vi "Do_ADAM_channel.vi"(4 "Scan Period":dbl format="%.2f", 5 "Previous Scan Value":dbl format="%.2f", 6 "Present scan array":dbl[](array[numeric]) format="%.2f", 7 "Value to Output":dbl format="%.2f", 8 "Ch Description":T1 {"Duty" format="%.0b"; "D" format="%#_5g"; "C" format="%#_5g"; "B" format="%#_5g"; "A" format="%#_5g"}, 9 "Ch names":string[](array[string])) -> (0 "Scan comment":string, 1 "Output":dbl format="%.3f")   [LabVIEW 2013]
uses:
  ADAM Client/Sub VIs/ADAM Controls/Ch_description_ADAM.ctl
  ADAM Client/Sub VIs/ADAM Controls/Module_type_ADAM.ctl
  ADAM Client/Sub VIs/ADAM Controls/Function_ADAM.ctl
  ADAM Client/Sub VIs/ADAM Controls/Channel_State.ctl
  ADAM Client/Sub VIs/ADAM Controls/Calib_type_ADAM.ctl
  ADAM Client/Sub VIs/ADAM Controls/Address.ctl
  ADAM Serial/Instrument drivers/Arduino/ctls_and_globals/Arduino tx msg cluster.ctl
  ADAM Client/Sub VIs/ADAM Controls/Remember_value_mode.ctl
  ADAM Client/Sub VIs/ADAM Controls/Search_mode.ctl
  Anemometry/Anemometry Sub Vis/Controls/In_Range.ctl
  Anemometry/Anemometry Sub Vis/Globals/Gas_management_global.vi
  ADAM_Global.vi
  Anemometry/Anemometry Sub Vis/Globals/Constants_global.vi
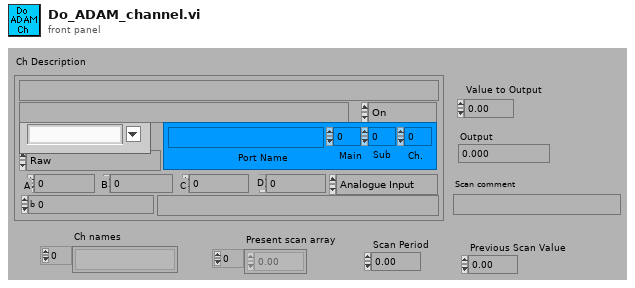
[diagram p1: front panel]
types:
  T1 = typedef "Ch_description_ADAM.ctl" = cluster{"Ch Name":string, "Type":T2, "Function":T3, "Ch State":T4, "Calibration type":T5, "A":dbl, "B":dbl, "C":dbl, "D":dbl, "Comments":string, "Address":T6, "String":string, "Duty":u16}
  T2 = typedef "Module_type_ADAM.ctl" = string
  T3 = typedef "Function_ADAM.ctl" = enum16{"Analogue Input", "Digital Input", "Event counter", "Event rate", "Analogue Output", "Digital Output", "Relay Output"}
  T4 = typedef "Channel_State.ctl" = enum16{"On", "Off", "Always On", "Always Off"}
  T5 = typedef "Calib_type_ADAM.ctl" = enum16{"Raw", "Bx + A", "Cx^2 + Bx + A", "Dx^3 + Cx^2 + Bx + A", "In Band", "Hi-Tec Q", "Hi-Tec M_dot", "Text"}
  T6 = typedef "Address.ctl" = cluster{"Main":i32, "Ch.":i32, "Sub":i32, "Port Name":string}
  T7 = typedef "Remember_value_mode.ctl" = enum16{"Read only", "Read and Write"}
  T8 = typedef "Search_mode.ctl" = enum16{"Between times", "All Times"}
  T9 = typedef "In_Range.ctl" = enum16{"%", "±", "% & ±"}
  T10 = typedef "Arduino tx msg cluster.ctl" = cluster{"dest":u8, "A/D":string, "R/W":string, "chan":u8, "val (float)":sgl}
  T11 = typedef "Valco_valve_ph.ctl" = u16
  T12 = cluster{"Centre Times":dbl[], "Output array":dbl[]}
  T13 = cluster{"Centre Times":dbl[], "Output array":dbl[]}[]
  T14 = typedef "LVDateTimeRec.ctl" = cluster{"fractional second":dbl, "second":i32, "minute":i32, "hour":i32, "day of month":i32, "month":i32, "year":i32, "day of week":i32, "day of year":i32, "DST":i32}
  T15 = typedef "Client_State_Cluster.ctl" = cluster{"Client Name":string, "Traverse level State":T16, "People to Email":string[], "Next Contact Time":dbl}
  T16 = typedef "Traverse_Level_State.ctl" = enum16{"Running", "Complete"}
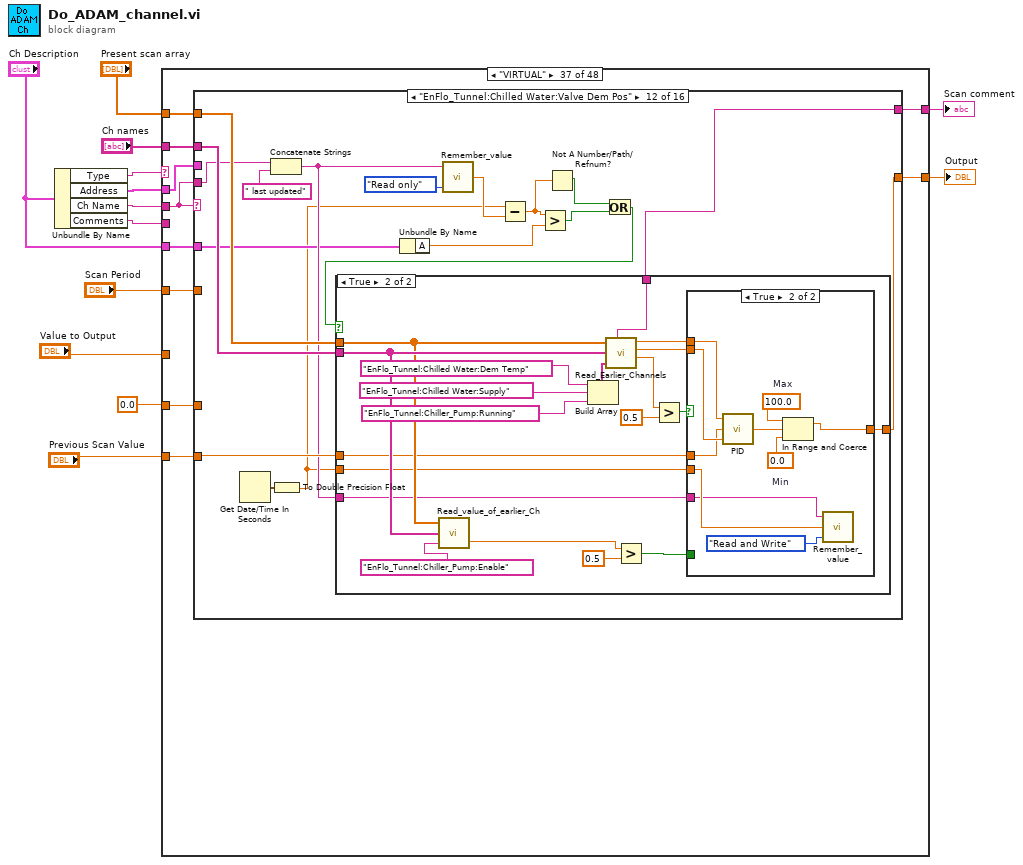
[diagram p0: block diagram]
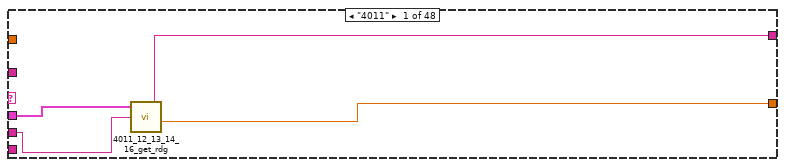
[diagram p2: hidden frame]
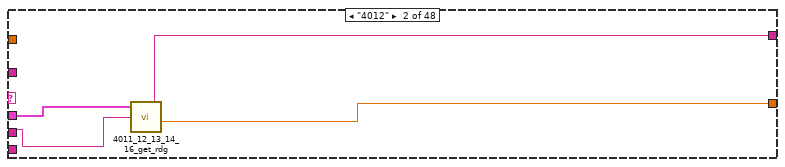
[diagram p3: hidden frame]
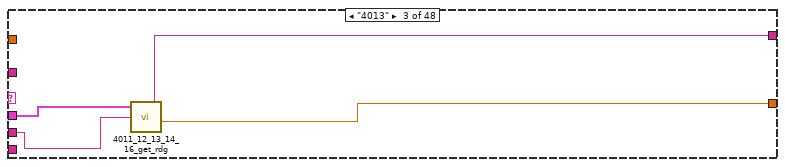
[diagram p4: hidden frame]
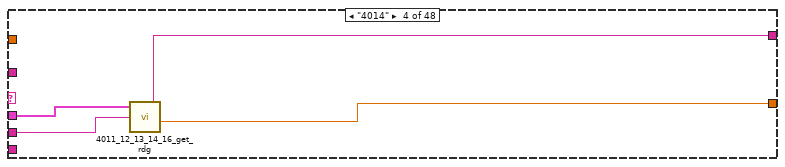
[diagram p5: hidden frame]
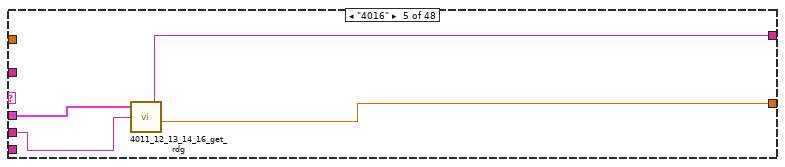
[diagram p6: hidden frame]
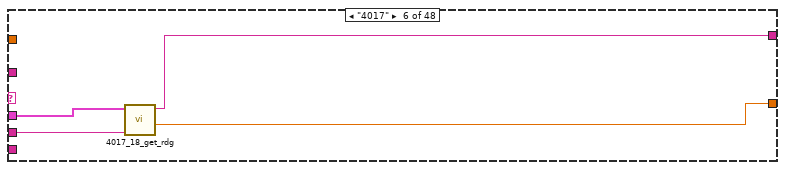
[diagram p7: hidden frame]
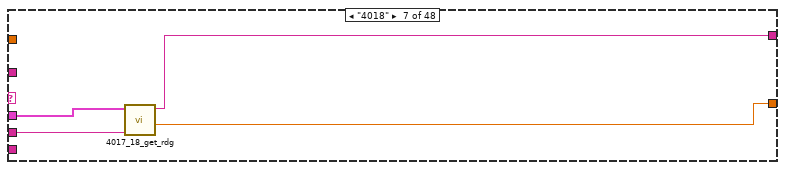
[diagram p8: hidden frame]
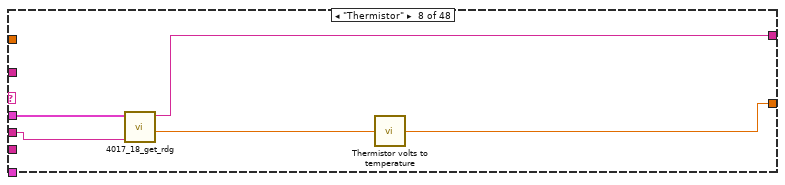
[diagram p9: hidden frame]
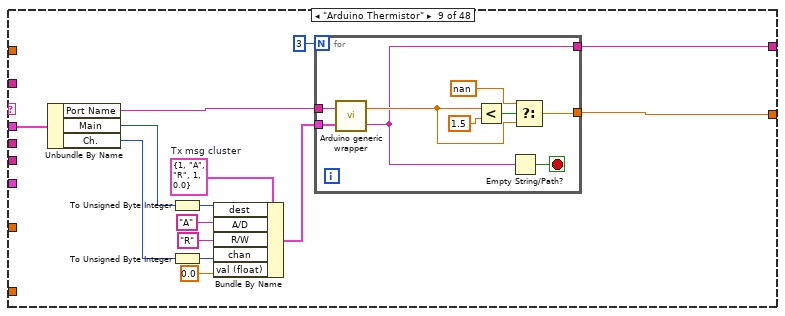
[diagram p10: hidden frame]
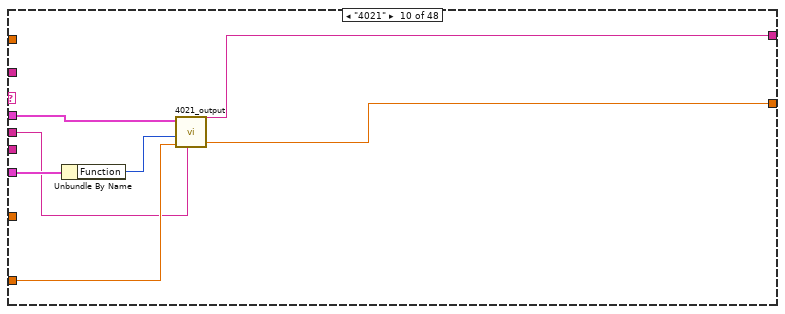
[diagram p11: hidden frame]
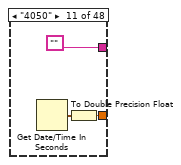
[diagram p12: hidden frame]
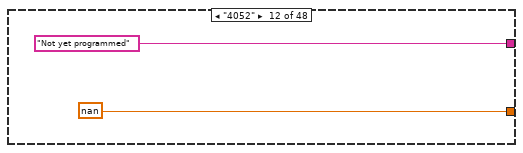
[diagram p13: hidden frame]
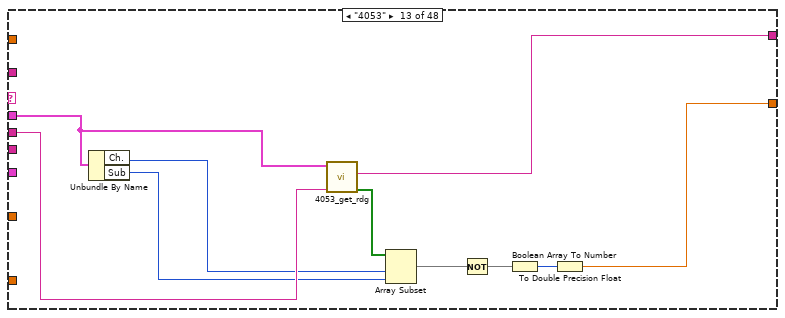
[diagram p14: hidden frame]
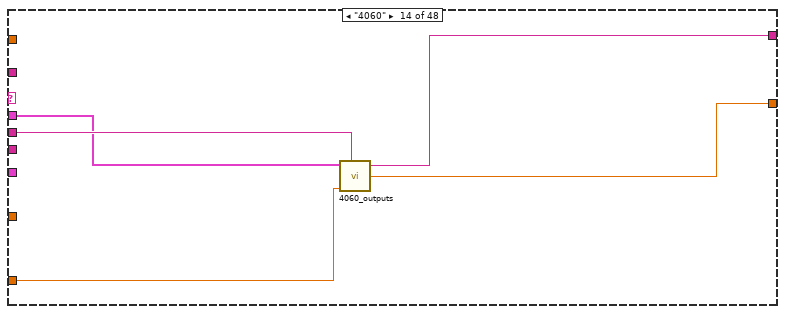
[diagram p15: hidden frame]
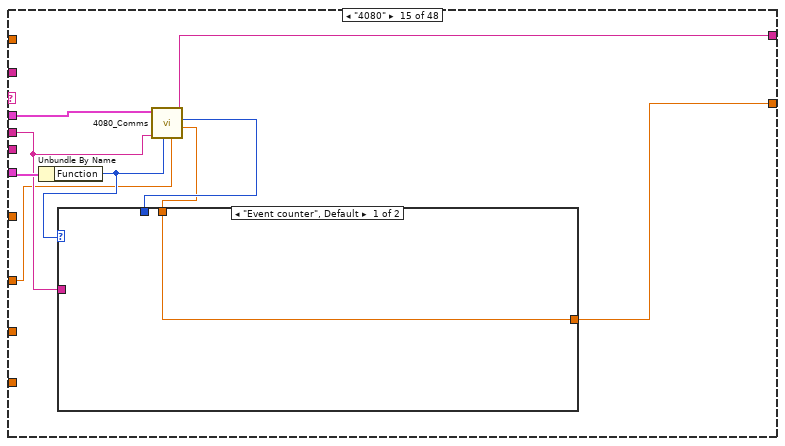
[diagram p16: hidden frame]
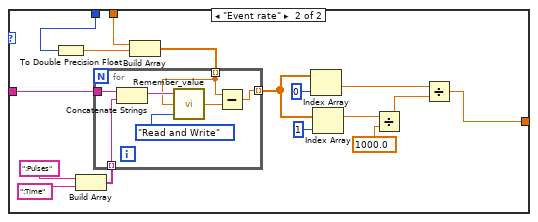
[diagram p17: hidden frame]
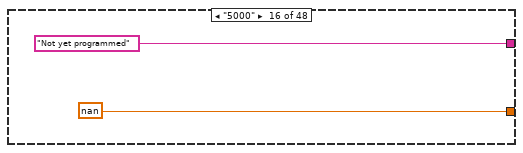
[diagram p18: hidden frame]
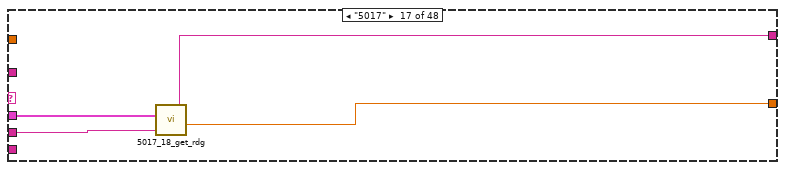
[diagram p19: hidden frame]
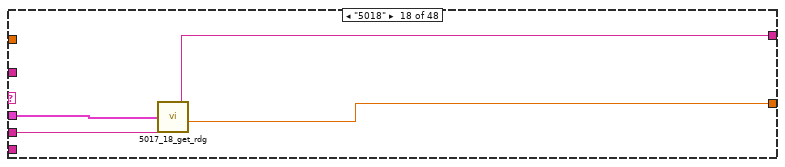
[diagram p20: hidden frame]
diagram:
  n1 = Unbundle By Name("Ch Description") -> ("Type"=w11:T2, "Address"=w10:T6, "Ch Name"=w2:string, "Comments"=w7:string)
  n2 = case shown="\"VIRTUAL\"" w11 {
    tunnel: [w16 w20 w24 w28 w32 w36 w40 w42 w48 w75 w78 nan w85 w94 w103 nan w133 w137 w142 w148 w156 w177 w199 w218 nan w286 w288 w304 w327 w366 nan w378 w409 w414 w415 w518 w542 w978 w980 w984 w989 w1001 w1035 w1061 w1071 w1076 w1086 0.0 ("Output")] -> w8
    tunnel: [w17 w21 w25 w29 w33 w37 w41 w46 w49 w76 "" "Not yet programmed" w90 w95 w105 "Not yet programmed" w134 w138 w145 w149 w155 w178 w200 w220 "Not yet programmed" w285 w289 w303 w319 w367 "Not yet programmed" w377 w410 w413 w436 w520 w541 "" "" w985 "" "" w1024 "" w1072 w1075 "Crazy time based random number!" "Warning; unmatched case in Do_ADAM_channel" ("Status note")] -> w5
    tunnel: w10 -> [w14 w18 w22 w26 w30 w34 w38 w44 w60 w70 _ _ w82 w93 w97 _ w135 w139 w146 w150 w154 w179 w201 w222 _ w283 w287 w306 w324 w372 _ _ w408 w411 _ _ w533 _ _ _ _ _ _ w1070 w1074 _ _ _]
    tunnel: "Ch Description" -> [_ _ _ _ _ _ _ _ _ w74 _ _ _ _ w104 _ _ _ _ _ w153 w176 w198 w221 _ _ _ _ _ _ _ w383 _ _ w441 _ w535 _ w981 w986 _ _ _ _ _ w1077 _ _]
    tunnel: w2 -> [w15 w19 w23 w27 w31 w35 w39 w45 _ w71 _ _ w91 w96 w100 _ w132 w136 w140 w147 w151 w173 w195 w219 _ w284 _ w305 w320 w371 _ _ _ w412 _ _ w538 _ _ _ _ w997 w1031 _ w1073 _ _ _]
    tunnel: "Ch names" -> [_ _ _ _ _ _ _ _ _ _ _ _ _ _ _ _ _ _ _ _ _ _ _ _ _ _ _ _ _ _ _ w384 _ _ w440 w525 w540 _ _ w987 _ _ _ _ _ _ _ _]
    tunnel: "Present scan array" -> [_ _ _ _ _ _ _ _ _ _ _ _ _ _ _ _ _ _ _ _ _ _ _ _ _ _ _ _ _ _ _ w381 _ _ w438 w524 w539 _ _ w988 _ _ _ _ _ _ _ _]
    tunnel: w7 -> [_ _ _ _ _ _ _ _ _ _ _ _ _ _ _ _ _ _ _ _ _ _ _ _ _ _ _ _ _ _ _ w376 _ _ w442 w523 _ _ _ _ _ _ _ _ _ _ _ _]
    tunnel: "Value to Output" -> [_ _ _ _ _ _ _ _ _ w72 _ _ _ w92 w98 _ _ _ w141 _ w152 w174 w196 w217 _ _ _ w302 w328 _ _ w382 _ _ _ _ _ _ _ _ _ _ _ w1065 _ _ _ _]
    tunnel: "Scan Period" -> [_ _ _ _ _ _ _ _ _ _ _ _ _ _ _ _ _ _ _ _ _ _ _ _ _ _ _ _ _ _ _ w379 _ _ _ _ w537 _ _ _ _ _ _ _ _ _ _ _]
    tunnel: "Previous Scan Value" -> [_ _ _ _ _ _ _ _ _ _ _ _ _ _ _ _ _ _ _ _ _ _ _ _ _ _ _ _ _ _ _ w380 _ _ w416 _ w536 w978 _ _ w989 _ _ _ _ _ _ _]
    tunnel: 0.0 -> [_ _ _ _ _ _ _ _ _ _ _ _ _ _ _ _ _ _ _ _ _ _ _ _ _ _ _ _ _ _ _ _ _ _ _ _ w534 _ _ _ _ _ _ _ _ _ _ _]
    frame "4011" {
      n3 = call "4011_12_13_14_16_get_rdg.vi"("Address"=w14, "Channel Name"=w15) -> ("Comment"=w17:string, "Reading"=w16:dbl)  [unwired: 1 in, 2 out]
    }
    frame "4012" {
      n4 = call "4011_12_13_14_16_get_rdg.vi"("Address"=w18, "Channel Name"=w19) -> ("Comment"=w21:string, "Reading"=w20:dbl)  [unwired: 1 in, 2 out]
    }
    frame "4013" {
      n5 = call "4011_12_13_14_16_get_rdg.vi"("Address"=w22, "Channel Name"=w23) -> ("Comment"=w25:string, "Reading"=w24:dbl)  [unwired: 1 in, 2 out]
    }
    frame "4014" {
      n6 = call "4011_12_13_14_16_get_rdg.vi"("Address"=w26, "Channel Name"=w27) -> ("Comment"=w29:string, "Reading"=w28:dbl)  [unwired: 1 in, 2 out]
    }
    frame "4016" {
      n7 = call "4011_12_13_14_16_get_rdg.vi"("Address"=w30, "Channel Name"=w31) -> ("Comment"=w33:string, "Reading"=w32:dbl)  [unwired: 1 in, 2 out]
    }
    frame "4017" {
      n8 = call "4017_18_get_rdg.vi"("Channel Name"=w35, "Address"=w34) -> ("Reading"=w36:dbl, "Comment"=w37:string)  [unwired: 2 in, 2 out]
    }
    frame "4018" {
      n9 = call "4017_18_get_rdg.vi"("Channel Name"=w39, "Address"=w38) -> ("Reading"=w40:dbl, "Comment"=w41:string)  [unwired: 2 in, 2 out]
    }
    frame "Thermistor" {
      n10 = call "4017_18_get_rdg.vi"("Channel Name"=w45, "Address"=w44) -> ("Reading"=w43:dbl, "Comment"=w46:string)  [unwired: 2 in, 2 out]
      n11 = call "Thermistor volts to temperature.vi"("V2 (V)"=w43) -> ("Temperature (degC)"=w42:dbl)
    }
    frame "Arduino Thermistor" {
      w54 = T10 {"dest"=1, "A/D"="A", "R/W"="R", "chan"=1, "val (float)"=0.0}  # Tx msg cluster
      n12 = Unbundle By Name(w60) -> ("Port Name"=w51:string, "Main"=w52:i32, "Ch."=w53:i32)
      n13 = To Unsigned Byte Integer(number=w52) -> (unsigned 8bit integer=w59:u8)
      n14 = To Unsigned Byte Integer(number=w53) -> (unsigned 8bit integer=w57:u8)
      n15 = Bundle By Name(cluster=w54, "dest"=w59, "A/D"="A", "R/W"="R", "chan"=w57, "val (float)"=sgl 0.0) -> (w50:T10)
      n16 = for {
        N: 3 -> [_]
        tunnel: w51 -> [w69]
        tunnel: w50 -> [w68]
        tunnel: [w61] -> w49
        tunnel: [w67] -> w48
        stop <- w62 stop-if-true
        n17 = call "Arduino generic wrapper.vi"("Tx msg cluster"=w68, "Port name"=w69) -> ("Scan comment"=w61:string, "Output"=w66:dbl)
        n18 = Less?(x=w66, y=1.5) -> (x < y?=w64:bool)
        n19 = Empty String/Path?(string/path=w61) -> (empty?=w62:bool)
        n20 = Select(t=nan ("f"), s=w64, f=w66) -> (s? t:f=w67:dbl)
      }
    }
    frame "4021" {
      n21 = Unbundle By Name(w74) -> ("Function"=w73:T3)
      n22 = call "4021_output.vi"("Address"=w70, "Function"=w73, "Set to:"=w72, "Channel Name"=w71) -> ("Comment"=w76:string, "Reading"=w75:dbl)  [unwired: 1 in, 1 out]
    }
    frame "4050" {
      n23 = Get Date/Time In Seconds() -> (seconds since 1Jan1904=w77:timestamp)
      n24 = To Double Precision Float(number=w77) -> (double precision float=w78:dbl)
    }
    frame "4052" {
    }
    frame "4053" {
      n25 = Unbundle By Name(w82) -> ("Ch."=w83:i32, "Sub"=w89:i32)
      n26 = call "4053_get_rdg.vi"("Channel Name"=w91, "Address"=w82) -> ("Boolean array"=w88:bool[], "Comment"=w90:string)  [unwired: 2 in, 2 out]
      n27 = Array Subset(array=w88, index=w83, length=w89) -> (w87:bool[])
      n28 = Not(x=w87) -> (.not. x?=w84:bool[])
      n29 = Boolean Array To Number(Boolean array=w84) -> (number=w86:u32)
      n30 = To Double Precision Float(number=w86) -> (double precision float=w85:dbl)
    }
    frame "4060" {
      n31 = call "4060_outputs.vi"("Address"=w93, "Value to Output"=w92, "Channel Name"=w96) -> ("Comment"=w95:string, "Reading"=w94:dbl)  [unwired: 2 in, 1 out]
    }
    frame "4080" {
      n32 = Unbundle By Name(w104) -> ("Function"=w99:T3)
      n33 = call "4080_Comms.vi"("Value to display"=w98, "Function"=w99, "Channel Name"=w100, "Address"=w97) -> ("Reading"=w101:dbl, "millisecond timer value"=w102:u32, "Comment"=w105:string)  [unwired: 2 in, 1 out]
      n34 = case shown="\"Event counter\", Default" w99 {
        tunnel: w100 -> [_ w122]
        tunnel: w102 -> [_ w115]
        tunnel: [w106 w107] -> w103
        tunnel: w101 -> [w106 w116]
        frame "Event counter", Default {
        }
        frame "Event rate" {
          n35 = To Double Precision Float(number=w115) -> (double precision float=w114:dbl)
          n36 = Build Array(":Pulses", ":Time") -> (w117:string[])
          n37 = Build Array(w116, w114) -> (w113:dbl[])
          n38 = for {
            tunnel: w122 -> [w126]
            tunnel: [w127] -> w110 mode=indexing
            tunnel: w117 -> [w124] mode=indexing
            tunnel: w113 -> [w123] mode=indexing
            n39 = Concatenate Strings(w126, w124) -> (w125:string)
            n40 = call "Remember_value.vi"("Mode"=Remember_value_mode."Read and Write", "Input Value"=w123, "Ch name"=w125) -> ("Output Value"=w128:dbl)
            n41 = Subtract(x=w123, y=w128) -> (x-y=w127:dbl)
          }
          n42 = Index Array(array=w110, index=0) -> (element=w108:dbl)
          n43 = Index Array(array=w110, index=1) -> (element=w109:dbl)
          n44 = Divide(x=w109, y=1000.0) -> (x/y=w120:dbl)
          n45 = Divide(x=w108, y=w120) -> (x/y=w107:dbl)
        }
      }
    }
    frame "5000" {
    }
    frame "5017" {
      n46 = call "5017_18_get_rdg.vi"("Address (all reqd.)"=w135, "Channel Name"=w132) -> ("Comment"=w134:string, "Reading"=w133:dbl)  [unwired: 3 out]
    }
    frame "5018" {
      n47 = call "5017_18_get_rdg.vi"("Address (all reqd.)"=w139, "Channel Name"=w136) -> ("Comment"=w138:string, "Reading"=w137:dbl)  [unwired: 3 out]
    }
    frame "5024" {
      n48 = call "5024_set_output.vi"("Set to:"=w141, "Address (all reqd.)"=w146, "Channel Name"=w140) -> ("Comment"=w145:string, "Good Reply"=w143:bool)  [unwired: 2 out]
      n49 = Select(t=w141, s=w143, f=nan) -> (s? t:f=w142:dbl)
    }
    frame "5051" {
      n50 = call "5051_56_get_inputs.vi"("Address (Main, Sub reqd.)"=w150, "Channel Name"=w147) -> ("Comment"=w149:string, "Single output"=w148:dbl)  [unwired: 3 out]
    }
    frame "5056" {
      n51 = Unbundle By Name(w153) -> ("Function"=w157:T3)
      n52 = case shown="\"Digital Input\"" w157 {
        tunnel: w154 -> [_ w163 w172]
        tunnel: ["This function is not available" w164 w170] -> w155
        tunnel: [nan ("A") w161 w167] -> w156
        tunnel: w152 -> [_ _ w166]
        tunnel: w151 -> [_ w160 w165]
        frame "Analogue Input", Default {
        }
        frame "Digital Input" {
          # "Readback value"
          n53 = call "5060_check_outputs.vi"("Address (Main, Sub reqd.)"=w163, "Channel Name"=w160) -> ("Comment"=w164:string, "Single Channel"=w162:i16)  [unwired: 3 out]
          n54 = To Double Precision Float(number=w162) -> (double precision float=w161:dbl)
        }
        frame "Relay Output" {
          # "Sets single o/p channel"
          n55 = Greater Than 0?(x=w166) -> (x > 0?=w171:bool)
          n56 = call "5056_60_set_single_output.vi"("Channel Name"=w165, "Address (all reqd.)"=w172, "Set state:"=w171) -> ("Comment"=w170:string, "Good Reply"=w169:bool)  [unwired: 2 out]
          n57 = Select(t=w166, s=w169, f=nan) -> (s? t:f=w167:dbl)
        }
      }
    }
    frame "5060" {
      n58 = Unbundle By Name(w176) -> ("Function"=w175:T3)
      n59 = case shown="\"Relay Output\"" w175 {
        tunnel: w179 -> [_ w185 w194]
        tunnel: ["This function is not available" w186 w192] -> w178
        tunnel: [nan ("A") w183 w189] -> w177
        tunnel: w174 -> [_ _ w188]
        tunnel: w173 -> [_ w182 w187]
        frame "Analogue Input", Default {
        }
        frame "Digital Input" {
          # "Readback value"
          n60 = call "5060_check_outputs.vi"("Address (Main, Sub reqd.)"=w185, "Channel Name"=w182) -> ("Comment"=w186:string, "Single Channel"=w184:i16)  [unwired: 3 out]
          n61 = To Double Precision Float(number=w184) -> (double precision float=w183:dbl)
        }
        frame "Relay Output" {
          # "Sets single o/p channel"
          n62 = Greater Than 0?(x=w188) -> (x > 0?=w193:bool)
          n63 = call "5056_60_set_single_output.vi"("Channel Name"=w187, "Address (all reqd.)"=w194, "Set state:"=w193) -> ("Comment"=w192:string, "Good Reply"=w191:bool)  [unwired: 2 out]
          n64 = Select(t=w188, s=w191, f=nan) -> (s? t:f=w189:dbl)
        }
      }
    }
    frame "6060" {
      n65 = Unbundle By Name(w198) -> ("Function"=w197:T3)
      n66 = case shown="\"Digital Input\"" w197 {
        tunnel: w201 -> [_ w207 w216]
        tunnel: ["This function is not available" w208 w214] -> w200
        tunnel: [nan ("A") w205 w211] -> w199
        tunnel: w196 -> [_ _ w210]
        tunnel: w195 -> [_ w204 w209]
        frame "Analogue Input", Default {
        }
        frame "Digital Input" {
          n67 = call "6060_read_all_I-O.vi"("Address (Main, Sub reqd.)"=w207, "Channel Name"=w204) -> ("Comment"=w208:string, "Single Input Channel"=w206:i16)  [unwired: 3 out]
          n68 = To Double Precision Float(number=w206) -> (double precision float=w205:dbl)
        }
        frame "Relay Output" {
          # "Sets single o/p channel"
          n69 = Greater Than 0?(x=w210) -> (x > 0?=w215:bool)
          n70 = call "6060_set_single_output.vi"("Channel Name"=w209, "Address (Main, Ch requd.)"=w216, "Set state:"=w215) -> ("Comment"=w214:string, "Good Reply"=w213:bool)  [unwired: 2 out]
          n71 = Select(t=w210, s=w213, f=nan) -> (s? t:f=w211:dbl)
        }
      }
    }
    frame "Tracker" {
      n72 = while {
        tunnel: w222 -> [w246]
        tunnel: w221 -> [w245]
        tunnel: [w239] -> w220
        tunnel: w219 -> [w238]
        tunnel: [w232] -> w218
        tunnel: w217 -> [w231]
        i -> [w228]
        stop <- w225 continue-if-true
        n73 = Unbundle By Name(w245) -> ("Function"=w244:T3)
        n74 = Unbundle By Name(w246) -> ("Port Name"=w243:string, "Ch."=w234:i32, "Main"=w242:i32, "Sub"=w241:i32)
        n75 = case shown="\"Analogue Output\"" w244 {
          tunnel: [enum16{"Set", "Read"}."Set" ("Set") enum16{"Set", "Read"}."Set" ("Set") enum16{"Set", "Read"}."Set" ("Set") enum16{"Set", "Read"}."Set" ("Set") enum16{"Set", "Read"}."Set" ("Set") enum16{"Set", "Read"}."Read" ("Set") enum16{"Set", "Read"}."Read" ("Set")] -> w229
          tunnel: [enum16{"Logic", "Analogue"}."Analogue" ("Analogue") enum16{"Logic", "Analogue"}."Logic" ("Analogue") enum16{"Logic", "Analogue"}."Logic" ("Analogue") enum16{"Logic", "Analogue"}."Logic" ("Analogue") enum16{"Logic", "Analogue"}."Logic" ("Analogue") enum16{"Logic", "Analogue"}."Logic" ("Analogue") enum16{"Logic", "Analogue"}."Analogue" ("Analogue")] -> w240
          frame "Analogue Output" {
          }
          frame "Digital Output" {
          }
          frame "Relay Output" {
          }
          frame "Event rate" {
          }
          frame "Event counter" {
          }
          frame "Digital Input" {
          }
          frame "Analogue Input" {
          }
        }
        n76 = call "TalkTracker.vi"("PORT NAME"=w243, "Set"=w229, "Channel Name"=w238, "Value to set"=w231, "MODULE ADDRESS"=w242, "LOCATION"=w234, "NO. LOCATIONS"=w241, "Analogue"=w240) -> ("Response"=w236:string, "Good Set?"=w223:bool, "Comment out"=w239:string)  [unwired: 1 in, 4 out]
        n77 = Match Pattern(string=w236, regular expression="\r\n") -> (before substring=w235:string)  [unwired: 4 out]
        n78 = case shown="\"Set\"" w229 {
          tunnel: w235 -> [_ w258]
          tunnel: [w250 w257] -> w233
          tunnel: w231 -> [w252 _]
          tunnel: nan ("Reading") -> [w251 w256]
          tunnel: [w249 w254] -> w226
          tunnel: [0 ("y") 1 ("y")] -> w224
          tunnel: w223 -> [w247 _]
          frame "Set" {
            n79 = Not(x=w247) -> (.not. x?=w249:bool)
            n80 = Select(t=w252, s=w247, f=w251) -> (s? t:f=w250:dbl)
          }
          frame "Read" {
            n81 = String Length(string=w258) -> (length=w260:i32)
            n82 = Fract/Exp String To Number(string=w258, default (0 dbl)=w256) -> (offset past number=w261:i32, number=w259:dbl)  [unwired: 2 out]
            n83 = Equal?(x=w260, y=w261) -> (x = y?=w255:bool)
            n84 = Not(x=w255) -> (.not. x?=w254:bool)
            n85 = Select(t=w259, s=w255, f=w256) -> (s? t:f=w257:dbl)
          }
        }
        n86 = case shown="0, Default" w234 {
          tunnel: w233 -> [w262 w265]
          tunnel: [w262 w263] -> w232
          frame 0, Default {
          }
          frame 283 {
            n87 = Equal To 0?(x=w265) -> (x = 0?=w266:bool)
            n88 = Select(t=nan ("Reading"), s=w266, f=w265) -> (s? t:f=w263:dbl)
          }
        }
        n89 = Less?(x=w228, y=w224) -> (x < y?=w227:bool)
        n90 = And(x=w226, y=w227) -> (x .and. y?=w225:bool)
      }
    }
    frame "WEST" {
    }
    frame "GILL" {
      n91 = call "Gill_get_rdg.vi"("Channel Name"=w284, "Address"=w283) -> ("Output"=w286:dbl, "Status note"=w285:string)  [unwired: 2 in, 2 out]
    }
    frame "ClimatronicsUDP" {
      n92 = call "ClimatronicsUDP_get_rdg.vi"("Address"=w287) -> ("Output"=w288:dbl, "Status note"=w289:string)  [unwired: 5 in]
    }
    frame "JEM" {
      n93 = Unbundle By Name(w306) -> ("Main"=w292:i32, "Ch."=w291:i32, "Port Name"=w301:string)
      n94 = case shown="0, Default" w291 {
        tunnel: [i16[] [-3, -2, -1, 0, 14, 29, 43, 57, 71, 86, 100] i16[] [0, 20, 40, 60, 80, 100, 120]] -> w295
        tunnel: [u8[] [10, 50, 80, 100, 120, 140, 160, 180, 200, 220, 240] u8[] [20, 50, 90, 130, 160, 200, 230]] -> w296
        frame 0, Default {
        }
        frame 1 {
        }
      }
      n95 = Add(x=w292, y=w291) -> (x+y=w290:i32)
      n96 = Threshold 1D Array(2:w302, 3:w295) -> (0:w298:dbl)  [unwired: 1 out]
      n97 = Round To Nearest(number=w298) -> (nearest integer value=w299:dbl)
      n98 = To Long Integer(number=w299) -> (32bit integer=w297:i32)
      n99 = Index Array(array=w296, index=w297) -> (element=w294:u8)
      n100 = call "DMX.vi"("Port Name"=w301, "DMX channel no."=w290, "Set value:"=w294, "Channel Name"=w305) -> ("error"=w300:bool)  [unwired: 2 out]
      n101 = Index Array(array=w295, index=w297) -> (element=w293:i16)
      n102 = case shown="False" w300 {
        tunnel: [w307 nan] -> w304
        tunnel: ["" "Comms Error"] -> w303
        tunnel: w293 -> [w309 _]
        frame False {
          n103 = To Double Precision Float(number=w309) -> (double precision float=w307:dbl)
        }
        frame True {
        }
      }
    }
    frame "VICI" {
      n104 = To Long Integer(number=w328) -> (32bit integer=w323:i32)
      n105 = Unbundle By Name(w324) -> ("Port Name"=w326:string, "Ch."=w325:i32)
      n106 = call "Valco_Valve_Position.vi"("Channel Name"=w320, "Valve Number"=w325, "Port Name"=w326, "Requested Posn."=w323) -> ("Error Message"=w318:string, "Achieved Posn."=w321:T11)  [unwired: 2 out]
      n107 = Empty String/Path?(string/path=w318) -> ()  [unwired: 1 out]
      n108 = case shown="True" TRUE {
        tunnel: w324 -> [w335 _]
        tunnel: w323 -> [w334 _]
        tunnel: [w333 w365] -> w322
        tunnel: w321 -> [_ w365]
        tunnel: w320 -> [w332 _]
        tunnel: [w331 w364] -> w319
        tunnel: w318 -> [_ w364]
        tunnel: w318 -> [w330 _]
        tunnel: "X10" ("Port Name") -> [w329 _]
        frame False {
          n109 = stacked-sequence {
            tunnel: w335 -> [_ _ _ _ _ w356]
            tunnel: w334 -> [_ _ _ _ _ w352]
            tunnel: [_ _ _ _ _ w355] -> w333
            tunnel: w332 -> [_ _ _ _ _ w354]
            tunnel: [_ _ _ _ _ w353] -> w331
            tunnel: w330 -> [_ w341 _ _ _ _]
            tunnel: w329 -> [w336 _ _ w344 _ _]
            frame #0 {
              w338 = 3 items=["-----", "A", "B", "C", "D", "E", "F", "G", "H", "I", "J", "K", "L", "M", "N", "O", "P"] ("House Code")
              n110 = call "X10control.vi"("Port Name"=w336, "Power Request (ON)"=FALSE, "House Code"=w338, "Unit No."=5) -> ()  [unwired: 6 out]
            }
            frame #1 {
              n111 = call "Server_Emails.vi"("Message"=w341, "Contact All clients?"=TRUE, "Subject"="Powering Down FID Valve" ("Error Type")) -> ()  [unwired: 2 in, 3 out]
            }
            frame #2 {
              n112 = Wait (ms)(milliseconds to wait=u32 20000) -> ()  [unwired: 1 out]
            }
            frame #3 {
              w346 = 3 items=["-----", "A", "B", "C", "D", "E", "F", "G", "H", "I", "J", "K", "L", "M", "N", "O", "P"] ("House Code")
              n113 = call "X10control.vi"("Port Name"=w344, "Power Request (ON)"=TRUE, "House Code"=w346, "Unit No."=5) -> ()  [unwired: 6 out]
            }
            frame #4 {
              n114 = Wait (ms)(milliseconds to wait=u32 5000) -> ()  [unwired: 1 out]
            }
            frame #5 {
              n115 = Build Array(1 ("element"), 2 ("element"), w352) -> (w349:i32[])
              n116 = for {
                tunnel: w356 -> [w361]
                tunnel: [w360] -> w355
                tunnel: w354 -> [w359]
                tunnel: [w358] -> w353
                tunnel: w349 -> [w357] mode=indexing
                n117 = Unbundle By Name(w361) -> ("Port Name"=w362:string, "Ch."=w363:i32)
                n118 = call "Valco_Valve_Position.vi"("Channel Name"=w359, "Valve Number"=w363, "Port Name"=w362, "Requested Posn."=w357) -> ("Error Message"=w358:string, "Achieved Posn."=w360:T11)  [unwired: 2 out]
              }
            }
          }
        }
        frame True {
        }
      }
      n119 = To Double Precision Float(number=w322) -> (double precision float=w327:dbl)
    }
    frame "Vaisala" {
      n120 = Unbundle By Name(w372) -> ("Main"=w368:i32, "Ch."=w369:i32, "Port Name"=w370:string)
      n121 = call "HMP231.vi"("Channel Name"=w371, "Port Name"=w370, "Channel"=w369, "Address"=w368) -> ("Output"=w366:dbl, "Status note"=w367:string)  [unwired: 2 out]
    }
    frame "DRUCK" {
    }
    frame "Run VI Named:" {
      n122 = Current VI's Path() -> (path=w393:path)
      n123 = Strip Path(path=w393) -> (stripped path=w394:path)  [unwired: 1 out]
      n124 = call <vilib>:"Trim Whitespace.vi"("string"=w376) -> ("trimmed string"=w375:string)  [unwired: 1 in]
      n125 = Strip Path(path=w394) -> (stripped path=w395:path)  [unwired: 1 out]
      n126 = Build Path(base path=w395, name or relative path="Run_vi_named") -> (appended path=w397:path)
      n127 = Build Path(base path=w397, name or relative path=w375) -> (appended path=w392:path)
      n128 = Open VI Reference(type specifier VI Refnum (for type only)=refnum<vi> refnum, vi path=w392) -> (vi reference=w388:refnum<vi>, error out=w387:errorcluster)  [unwired: 1 in, 3 out]
      n129 = property class="VI Interface Type 0"(reference=w388, error in=w387) -> (reference out=w390:refnum<vi>, error out=w389:errorcluster, "Front Panel Window:Open"=w391:bool)
      n130 = case shown="False" w391 {
        tunnel: w390 -> [w405 w407]
        tunnel: w389 -> [w404 w406]
        tunnel: [w403 w407] -> w386
        tunnel: [w401 w406] -> w385
        frame False {
          n131 = property class="VI Interface Type 0"(reference=w405, error in=w404, "Front Panel Window:Open"=TRUE) -> (reference out=w403:refnum<vi>, error out=w401:errorcluster)
        }
        frame True {
        }
      }
      n132 = call-by-ref "?"(reference=w386, error in=w385, "Scan Period"=w379, "Previous Scan Value"=w380, "Present scan array"=w381, "Value to Output"=w382, "Ch Description"=w383, "Ch names"=w384) -> (reference out=w399:refnum<vi>, error out=w400:errorcluster, "Scan comment"=w377:string, "Output"=w378:dbl)  [unwired: 2 in]
      n133 = Close Reference(reference=w399, error in (no error)=w400) -> ()  [unwired: 1 out]
    }
    frame "IR2100" {
      n134 = call "IR2100_get_rdg.vi"("Address"=w408) -> ("Comment"=w410:string, "Reading"=w409:dbl)  [unwired: 2 in, 2 out]
    }
    frame "PPT" {
      n135 = call "PPT_get_rdg.vi"("Channel Name"=w412, "Address"=w411) -> ("Reading"=w414:dbl, "Comment"=w413:string)  [unwired: 2 in, 2 out]
    }
    frame "Comparator" {
      # "A Warn if above this value\nB Warn if below this value\nC  Hysteresis margin\nD is the averaging time in minutes\nComments   is Channel name to check"
      n136 = Unbundle By Name(w441) -> ("D"=w424:dbl)
      n137 = Match Pattern(string=w442, regular expression=":::" ("String to match")) -> (before substring=w439:string)  [unwired: 4 out]
      n138 = call "Read_value_of_earlier_Ch.vi"("Desired Ch to Read"=w439, "Ch names"=w440, "Present scan array"=w438) -> ("Value"=w423:dbl, "Scan comment"=w437:string)  [unwired: 1 in]
      n139 = Equal?(x=w416, y=1.0) -> (x = y?=w432:bool)
      n140 = Unbundle By Name(w441) -> ("A"=w435:dbl, "B"=w434:dbl, "C"=w433:dbl)
      n141 = Equal To 0?(x=w424) -> (x = 0?=w422:bool)
      n142 = case shown="True" w432 {
        tunnel: [w448 w453] -> w430
        tunnel: w435 -> [w448 w452]
        tunnel: w434 -> [w447 w451]
        tunnel: [w447 w449] -> w431
        tunnel: w433 -> [_ w450]
        frame False {
        }
        frame True {
          n143 = Subtract(x=w452, y=w450) -> (x-y=w453:dbl)
          n144 = Add(x=w451, y=w450) -> (x+y=w449:dbl)
        }
      }
      n145 = case shown="False" w422 {
        tunnel: [w458 w461] -> w445
        tunnel: w439 -> [w460 _]
        tunnel: [w456 w462] -> w421
        tunnel: w424 -> [w454 _]
        tunnel: w423 -> [_ w462]
        tunnel: w437 -> [w458 w461]
        frame False {
          n146 = Build Array(w460) -> (w455:string[])
          n147 = call "Get_Channel_averages.vi"("Desired Ch Names"=w455, "Averaging time (mins)"=w454) -> ("number"=w457:dbl[])  [unwired: 1 in, 2 out]
          n148 = Index Array(array=w457, index=0) -> (element=w456:dbl)
        }
        frame True {
        }
      }
      n149 = Not(x=w432) -> (.not. x?=w425:bool)
      n150 = In Range and Coerce(upper limit=w430, x=w421, lower limit=w431) -> (In Range?=w426:bool)  [unwired: 1 out]
      n151 = Greater?(x=w421, y=w430) -> (0:w429:bool)
      n152 = Not A Number/Path/Refnum?(number/path/refnum=w421) -> (NaN/Path/Refnum?=w418:bool)
      n153 = Equal?(x=w426, y=w425) -> (x = y?=w420:bool)
      n154 = Or(x=w420, y=w418) -> (x .or. y?=w419:bool)
      n155 = case shown="False" w419 {
        tunnel: w439 -> [w469 _]
        tunnel: w430 -> [w468 _]
        tunnel: w441 -> [w467 _]
        tunnel: w431 -> [w466 _]
        tunnel: w426 -> [w465 _]
        tunnel: w421 -> [w464 _]
        tunnel: w429 -> [w463 _]
        frame False {
          n156 = stacked-sequence {
            seq-local: [w475 _ _ _ _] -> [_ _ _ w516 _]
            seq-local: [_ w495 _ _ _] -> [_ _ _ w513 _]
            seq-local: [w473 _ _ _ _] -> [_ _ _ w509 _]
            tunnel: w469 -> [w477 w503 _ w515 _]
            tunnel: w468 -> [w476 _ _ _ _]
            tunnel: w467 -> [_ _ w508 w517 _]
            tunnel: w466 -> [w474 _ _ _ _]
            tunnel: w465 -> [w472 _ _ _ _]
            tunnel: w464 -> [w471 _ _ _ _]
            tunnel: w463 -> [w470 _ _ _ _]
            frame #0 {
              n157 = case shown="True" w472 {
                tunnel: w477 -> [w482 w493]
                tunnel: w476 -> [_ w486]
                tunnel: [w480 w492] -> w475
                tunnel: w474 -> [_ w485]
                tunnel: ["OK " ""] -> w473
                tunnel: w471 -> [w478 _]
                tunnel: w470 -> [_ w483]
                frame True {
                  n158 = Format Into String(format string="The channel named %s is now  %.3f" ("Format String"), w482, w478) -> (resulting string=w480:string)  [unwired: 2 in, 1 out]
                }
                frame False {
                  n159 = Select(t=w486, s=w483, f=w485) -> (s? t:f=w484:dbl)
                  n160 = Select(t="greater", s=w483, f="less") -> (s? t:f=w488:string)
                  n161 = Format Into String(format string="%s is %s than %.3f" ("Format String"), w493, w488, w484) -> (resulting string=w492:string)  [unwired: 2 in, 1 out]
                }
              }
            }
            frame #1 {
              n162 = Build Array(w503) -> (w502:string[])
              n163 = call "Channel_Names_and_indicies.vi"("All Active Channels"=FALSE, "Desired Ch Names"=w502) -> ("Indicies"=w500:i32[])  [unwired: 1 out]
              n164 = call "Specified_Channels_server.vi"("Mode"=Search_mode."All Times", "Requested channels"=w500) -> ("Output array"=w498:dbl[][], "Centre Times"=w494:dbl[])  [unwired: 3 in, 3 out]
              n165 = Index Array(array=w498, index (row)=0) -> (element=w496:dbl[])  [unwired: 1 in]
              n166 = Bundle("Centre Times"=w494, "Output array"=w496) -> (w499:T12)  [unwired: 1 out]
              n167 = Build Array(w499) -> (w495:T13)
            }
            frame #2 {
              w506 = TRUE  # Contact All clients?
              n168 = Unbundle By Name(w508) -> ("String"=w507:string)
              n169 = call "Get_array_values_fr_String.vi"("String Value"=w507) -> ("String array"=w505:string[])  [unwired: 1 out]
              n170 = call "Client_email_addresses.vi"("Extra People to Email"=w505, "Contact All clients?"=w506) -> ()  [unwired: 1 in]
            }
            frame #3 {
              n171 = Unbundle By Name(w517) -> ("Ch Name"=w510:string)
              n172 = Build Array(w515) -> (w514:string[])
              n173 = Concatenate Strings(w509, w510) -> (w511:string)
              n174 = call "Email_Attachment_Plot.vi"("X axis name"="Time", "XY Graph"=w513, "Series Names"=w514, "message"=w516, "subject ([No Subject])"=w511) -> ()  [unwired: 1 in, 1 out]
            }
            frame #4 {
            }
          }
        }
        frame True {
        }
      }
      n175 = Concatenate Strings(w445, "") -> (w436:string)
      n176 = Select(t=0.0, s=w426, f=1.0) -> (s? t:f=w417:dbl)
      n177 = Select(t=w416, s=w418, f=w417) -> (s? t:f=w415:dbl)
    }
    frame "Average" {
      # "The Channel names to average must appear in the comments field separated by semi colons"
      n178 = call "Get_array_values_fr_String.vi"("String Value"=w523) -> ("String array"=w522:string[])  [unwired: 1 out]
      n179 = for {
        tunnel: w525 -> [w532]
        tunnel: w524 -> [w531]
        tunnel: w522 -> [w530] mode=indexing
        shift-right: [w527] -> w520
        shift-left: "" -> [w529]
        tunnel: [w526] -> w519 mode=indexing
        n180 = call "Read_value_of_earlier_Ch.vi"("Desired Ch to Read"=w530, "Ch names"=w532, "Present scan array"=w531) -> ("Value"=w526:dbl, "Scan comment"=w528:string)  [unwired: 1 in]
        n181 = Concatenate Strings(w529, w528) -> (w527:string)
      }
      n182 = call "Mean_fr_NaN_data.vi"("Data"=w519) -> ("Mean value"=w518:dbl)  [unwired: 1 out]
    }
    frame "VIRTUAL" {
      n183 = case shown="\"EnFlo_Tunnel:Chilled Water:Valve Dem Pos\"" w538 {
        tunnel: [w552 w566 w580 w602 w617 w628 w644 w675 w702 w737 w741 w775 w828 w854 w881 w901] -> w542
        tunnel: [w543 w572 w578 w606 w611 w626 w653 "" w706 w731 w747 w772 w827 w853 "" w902] -> w541
        tunnel: w540 -> [w549 w574 w584 w608 w613 w631 w655 w679 w708 w733 w749 w773 w833 w858 _ w904]
        tunnel: w539 -> [w550 w573 w585 w607 w612 w632 w654 w680 w709 w732 w748 w774 w835 w860 _ w903]
        tunnel: w538 -> [w547 _ _ _ _ _ _ _ _ _ _ w761 _ _ w876 _]
        tunnel: w537 -> [w548 _ _ _ _ _ _ _ _ _ _ _ w825 w852 w881 w900]
        tunnel: w536 -> [w551 _ _ _ _ _ _ _ _ _ _ w776 w829 w855 _ w899]
        tunnel: w535 -> [_ _ w576 _ _ _ _ _ _ _ _ w767 _ _ _ _]
        tunnel: w534 -> [_ w565 _ _ _ w625 _ _ _ _ _ _ _ _ _ _]
        tunnel: w533 -> [_ _ _ _ _ _ _ _ _ _ _ _ _ _ _ _]
        frame "GMU:Remaining:", Default {
          n184 = Match Pattern(string=w547, regular expression="GMU:Remaining:" ("String to match")) -> (match substring=w545:string)  [unwired: 4 out]
          n185 = Empty String/Path?(string/path=w545) -> (empty?=w544:bool)
          n186 = case shown="False" w544 {
            tunnel: [w559 nan] -> w552
            tunnel: w551 -> [w558 _]
            tunnel: w550 -> [w557 _]
            tunnel: w549 -> [w556 _]
            tunnel: w548 -> [w555 _]
            tunnel: w547 -> [w554 _]
            tunnel: [w553 w561] -> w543
            frame False {
              n187 = call "Update_Rem_gas.vi"("Scan Period (s)"=w555, "Gas Remaining in"=w558, "Ch name"=w554, "Ch names"=w556, "Present scan array"=w557) -> ("Gas Remaining out"=w559:dbl, "Comments"=w553:string)  [unwired: 1 out]
            }
            frame True {
              n188 = Current VI's Path() -> (path=w563:path)
              n189 = Path To String(path=w563) -> (string=w562:string)
              n190 = Concatenate Strings(" was not matched in ", w562) -> (w561:string)
            }
          }
        }
        frame "GMU:Source:Meas Q" {
          n191 = call "Calculate_Release_Flowrates.vi"("Ch names"=w574, "Units"=enum16{"Q l/min", "M_dot Kg/min"}."Q l/min", "Present scan array"=w573) -> ("Trace"=w570:dbl, "Carrier"=w571:dbl, "Scan comments"=w572:string)
          n192 = Add(x=w571, y=w570) -> (x+y=w567:dbl)
          n193 = Not Equal To 0?(x=w567) -> (x != 0?=w568:bool)
          n194 = Select(t=w567, s=w568, f=w565) -> (s? t:f=w566:dbl)
        }
        frame "GMU:Detector:Strength" {
          n195 = Unbundle By Name(w576) -> ("C"=w575:dbl)
          n196 = call "Read_value_of_earlier_Ch.vi"("Desired Ch to Read"="GMU:Detector:Meas Current", "Ch names"=w584, "Present scan array"=w585) -> ("Value"=w581:dbl, "Scan comment"=w579:string)  [unwired: 1 in]
          n197 = Greater?(x=w581, y=w575) -> (0:w582:bool)
          n198 = case shown="True" w582 {
            tunnel: w576 -> [_ w597]
            tunnel: w581 -> [_ w592]
            tunnel: [100.0 ("Eng Values") w590] -> w580
            tunnel: ["Fault" w593] -> w577
            frame False {
            }
            frame True {
              n199 = Unbundle By Name(w597) -> ("D"=w588:dbl, "A"=w596:dbl, "B"=w595:dbl)
              n200 = Less?(x=w592, y=w588) -> (x < y?=w591:bool)
              n201 = Build Array(w596, w595) -> (w594:dbl[])
              n202 = call "Polynomial_convert.vi"("Calib constants"=w594, "Voltage"=w592) -> ("Eng Values"=w589:dbl)  [unwired: 4 out]
              n203 = case shown="True" w591 {
                tunnel: ["Saturated" ""] -> w593
                tunnel: [100.0 ("Eng Values") w600] -> w590
                tunnel: w589 -> [_ w600]
                frame False {
                }
                frame True {
                }
              }
            }
          }
          n204 = Concatenate Strings(w579, w577) -> (w578:string)
        }
        frame "GMU:Source:Meas M_dot" {
          n205 = call "Calculate_Release_Flowrates.vi"("Ch names"=w608, "Units"=enum16{"Q l/min", "M_dot Kg/min"}."M_dot Kg/min", "Present scan array"=w607) -> ("Trace"=w604:dbl, "Carrier"=w605:dbl, "Scan comments"=w606:string)
          n206 = Add(x=w605, y=w604) -> (x+y=w602:dbl)
        }
        frame "GMU:Source:Meas Density" {
          n207 = Build Array("GMU:Source:Meas M_dot", "GMU:Source:Meas Q") -> (w614:string[])
          n208 = call "Read_Earlier_Channels.vi"("Present scan array"=w612, "Ch names"=w613, "Desired Channels"=w614) -> ("Scan comments"=w611:string, "Index 0"=w610:dbl, "Index 1"=w609:dbl)  [unwired: 3 out]
          n209 = Not Equal To 0?(x=w610) -> (x != 0?=w618:bool)
          n210 = case shown="False" w618 {
            tunnel: w610 -> [_ w622]
            tunnel: w609 -> [_ w621]
            tunnel: [0.0 w620] -> w617
            frame False {
            }
            frame True {
              n211 = Divide(x=w622, y=w621) -> (x/y=w623:dbl)
              n212 = Multiply(x=w623, y=1000.0) -> (x*y=w620:dbl)
            }
          }
        }
        frame "GMU:Source:Meas Den Ratio" {
          n213 = call "Read_value_of_earlier_Ch.vi"("Desired Ch to Read"="GMU:Source:Meas Density", "Ch names"=w631, "Present scan array"=w632) -> ("Value"=w627:dbl, "Scan comment"=w626:string)  [unwired: 1 in]
          n214 = Equal?(x=w627, y=w625) -> (x = y?=w629:bool)
          n215 = case shown="False" w629 {
            tunnel: w627 -> [w634 _]
            tunnel: [w633 w639] -> w628
            tunnel: w625 -> [_ w639]
            frame False {
              n216 = global read "Gas_management_global.vi" "Release temp (deg C)"() -> (w637:dbl)
              n217 = global read "Gas_management_global.vi" "Atmos Pres (mbars)"() -> (w636:dbl)
              n218 = call "Gas_Density.vi"("Pressure (mbars)"=w636, "Temperature (deg C)"=w637, "Gas Name"="Air") -> ("Density Kg/m3"=w635:dbl)
              n219 = Divide(x=w634, y=w635) -> (x/y=w633:dbl)
            }
            frame True {
            }
          }
        }
        frame "GMU:Source:Meas Strength" {
          n220 = call "Calculate_Release_Flowrates.vi"("Ch names"=w655, "Units"=enum16{"Q l/min", "M_dot Kg/min"}."Q l/min", "Present scan array"=w654) -> ("Trace"=w647:dbl, "Carrier"=w648:dbl, "Scan comments"=w653:string)
          n221 = Equal To 0?(x=w648) -> (x = 0?=w650:bool)
          n222 = Equal To 0?(x=w647) -> (x = 0?=w651:bool)
          n223 = And(x=w650, y=w651) -> (x .and. y?=w649:bool)
          n224 = case shown="False" w649 {
            tunnel: w648 -> [w666 _]
            tunnel: w647 -> [w665 _]
            tunnel: [w664 0.0] -> w643
            frame False {
              n225 = Add(x=w666, y=w665) -> (x+y=w669:dbl)
              n226 = Divide(x=w665, y=w669) -> (x/y=w668:dbl)
              n227 = Multiply(x=w668, y=100.0) -> (x*y=w664:dbl)
            }
            frame True {
            }
          }
          n228 = while {
            tunnel: [w657] -> w640
            tunnel: [w658] -> w642
            tunnel: w643 -> [w663]
            shift-left: _ -> [w657]
            shift-left: _ -> [w662]
            shift-right: [w663] -> _
            stop <- FALSE continue-if-true
            w661 = 6.0 ("y")
            n229 = Less?(x=w662, y=w661) -> (x < y?=w660:bool)
            n230 = Less?(x=w657, y=w661) -> (x < y?=w659:bool)
            n231 = Or(x=w660, y=w659) -> (x .or. y?=w658:bool)
          }
          n232 = Greater?(x=w643, y=7.0) -> (0:w641:bool)
          n233 = And(x=w642, y=w641) -> (x .and. y?=w645:bool)
          n234 = Select(t=w640, s=w645, f=w643) -> (s? t:f=w644:dbl)
        }
        frame "EnFlo_Tunnel:Temp:Inlet_Av" {
          w678 = 0.0 ("Value")
          w672 = "EnFlo_Tunnel:Temp:Inlet"
          n235 = String Length(string=w672) -> (length=w673:i32)
          n236 = for {
            tunnel: w680 -> [w686] mode=indexing
            tunnel: w679 -> [w685] mode=indexing
            shift-right: [w693] -> w677
            shift-left: w678 -> [w692]
            shift-right: [w690] -> w676
            shift-left: w678 -> [w691]
            tunnel: w673 -> [w689]
            tunnel: w672 -> [w687]
            tunnel: "EnFlo_Tunnel:Temp:Inlet_Av" -> [w684]
            n237 = String Subset(string=w685, length (rest)=w689) -> (substring=w688:string)  [unwired: 1 out]
            n238 = Equal?(x=w688, y=w687) -> (x = y?=w682:bool)
            n239 = Not Equal?(x=w685, y=w684) -> (x != y?=w683:bool)
            n240 = And(x=w682, y=w683) -> (x .and. y?=w681:bool)
            n241 = case shown="True" w681 {
              tunnel: [w695 w699] -> w693
              tunnel: w692 -> [w695 w700]
              tunnel: w686 -> [_ w698]
              tunnel: w691 -> [w694 w697]
              tunnel: [w694 w696] -> w690
              frame False {
              }
              frame True {
                n242 = Add(x=w698, y=w700) -> (x+y=w699:dbl)
                n243 = Increment(x=w697) -> (x+1=w696:dbl)
              }
            }
          }
          n244 = Divide(x=w677, y=w676) -> (x/y=w675:dbl)
        }
        frame "EnFlo Lab:labstrat1:Av Temp" {
          w705 = 0.0 ("Value")
          n245 = for {
            tunnel: w709 -> [w721]
            tunnel: w708 -> [w720]
            shift-right: [w717] -> w706
            shift-left: "" -> [w718]
            shift-right: [w715] -> w704
            shift-left: w705 -> [w714]
            shift-right: [w711] -> w703
            shift-left: w705 -> [w712]
            tunnel: string[] ["EnFlo Lab:labstrat1:Z=4.5m", "EnFlo Lab:labstrat1:Z=3.5m", "EnFlo Lab:labstrat1:Z=2.5m", "EnFlo Lab:labstrat1:Z=1.5m", "EnFlo Lab:labstrat1:Z=0.5m"] -> [w710] mode=indexing
            n246 = call "Read_value_of_earlier_Ch.vi"("Desired Ch to Read"=w710, "Ch names"=w720, "Present scan array"=w721) -> ("Value"=w713:dbl, "Scan comment"=w719:string)  [unwired: 1 in]
            n247 = Concatenate Strings(w718, w719) -> (w717:string)
            n248 = Not A Number/Path/Refnum?(number/path/refnum=w713) -> (NaN/Path/Refnum?=w716:bool)
            n249 = case shown="True" w716 {
              tunnel: [w725 w728] -> w715
              tunnel: w714 -> [w726 w728]
              tunnel: w713 -> [w724 _]
              tunnel: w712 -> [w723 w727]
              tunnel: [w722 w727] -> w711
              frame False {
                n250 = Add(x=w724, y=w726) -> (x+y=w725:dbl)
                n251 = Increment(x=w723) -> (x+1=w722:dbl)
              }
              frame True {
              }
            }
          }
          n252 = Divide(x=w704, y=w703) -> (x/y=w702:dbl)
        }
        frame "EnFlo Lab:labstrat1:Delta T" {
          n253 = Build Array("EnFlo Lab:labstrat1:Z=4.5m", "EnFlo Lab:labstrat1:Z=0.5m") -> (w736:string[])
          n254 = call "Read_Earlier_Channels.vi"("Present scan array"=w732, "Ch names"=w733, "Desired Channels"=w736) -> ("Scan comments"=w731:string, "Index 0"=w730:dbl, "Index 1"=w729:dbl)  [unwired: 3 out]
          n255 = Subtract(x=w730, y=w729) -> (x-y=w737:dbl)
        }
        frame "EnFlo_Tunnel:Inlet:K_Factor" {
          n256 = Build Array("EnFlo_Tunnel:Pressure:Static", "EnFlo_Tunnel:Reference:Velocity", "Froude:NPL:Atmos_Press", "EnFlo_Tunnel:Temp:Inlet_Av") -> (w752:string[])
          n257 = call "Read_Earlier_Channels.vi"("Present scan array"=w748, "Ch names"=w749, "Desired Channels"=w752) -> ("Scan comments"=w747:string, "Index 0"=w742:dbl, "Index 1"=w739:dbl, "Index 2"=w743:dbl, "Index 3"=w744:dbl)  [unwired: 1 out]
          n258 = Greater?(x=w739, y=0.8) -> (0:w740:bool)
          n259 = case shown="True" w740 {
            tunnel: w744 -> [_ w758]
            tunnel: w743 -> [_ w757]
            tunnel: w739 -> [_ w756]
            tunnel: w742 -> [_ w755]
            tunnel: [nan w754] -> w741
            frame False {
            }
            frame True {
              n260 = formula code="Rho=(Patmos*100)/(287*(T+273));\nDyn_Pres=0.5*Rho*U*U;\nK=(-Pstatic/Dyn_Pres)-1;"("Pstatic"=w755, "Patmos"=w757, "T"=w758, "U"=w756) -> ("K"=w754:dbl)  [unwired: 2 out]
            }
          }
        }
        frame "EnFlo_Tunnel:Chilled Water:Valve Dem Pos" {
          n261 = Get Date/Time In Seconds() -> (seconds since 1Jan1904=w760:timestamp)
          n262 = Concatenate Strings(w761, " last updated") -> (w769:string)
          n263 = To Double Precision Float(number=w760) -> (double precision float=w759:dbl)
          n264 = Unbundle By Name(w767) -> ("A"=w766:dbl)
          n265 = call "Remember_value.vi"("Mode"=Remember_value_mode."Read only", "Ch name"=w769) -> ("Output Value"=w768:dbl)  [unwired: 1 in]
          n266 = Subtract(x=w759, y=w768) -> (x-y=w765:dbl)
          n267 = Greater?(x=w765, y=w766) -> (0:w764:bool)
          n268 = Not A Number/Path/Refnum?(number/path/refnum=w765) -> (NaN/Path/Refnum?=w763:bool)
          n269 = Or(x=w763, y=w764) -> (x .or. y?=w762:bool)
          n270 = case shown="True" w762 {
            tunnel: w776 -> [w777 w779]
            tunnel: [w777 w796] -> w775
            tunnel: w774 -> [_ w788]
            tunnel: w773 -> [_ w789]
            tunnel: ["" w794] -> w772
            tunnel: w769 -> [_ w784]
            tunnel: w759 -> [_ w780]
            frame False {
            }
            frame True {
              n271 = call "Read_value_of_earlier_Ch.vi"("Desired Ch to Read"="EnFlo_Tunnel:Chiller_Pump:Enable", "Ch names"=w789, "Present scan array"=w788) -> ("Value"=w787:dbl)  [unwired: 1 in, 1 out]
              n272 = Build Array("EnFlo_Tunnel:Chilled Water:Dem Temp", "EnFlo_Tunnel:Chilled Water:Supply", "EnFlo_Tunnel:Chiller_Pump:Running") -> (w795:string[])
              n273 = call "Read_Earlier_Channels.vi"("Present scan array"=w788, "Ch names"=w789, "Desired Channels"=w795) -> ("Scan comments"=w794:string, "Index 0"=w793:dbl, "Index 1"=w792:dbl, "Index 2"=w782:dbl)  [unwired: 2 out]
              n274 = Greater?(x=w787, y=0.5) -> (0:w785:bool)
              n275 = Greater?(x=w782, y=0.5) -> (0:w781:bool)
              n276 = case shown="True" w781 {
                tunnel: [w811 w819] -> w796
                tunnel: w793 -> [_ w821]
                tunnel: w792 -> [_ w820]
                tunnel: w780 -> [_ w818]
                tunnel: w785 -> [w802 _]
                tunnel: w784 -> [_ w817]
                tunnel: w779 -> [_ w815]
                frame False {
                  n277 = Seconds To Date/Time() -> (date time rec=w799:T14)  [unwired: 2 out]
                  n278 = Unbundle By Name(w799) -> ("day of week"=w806:i32, "hour"=w808:i32)
                  n279 = Less?(x=w808, y=3) -> (x < y?=w803:bool)
                  n280 = Equal?(x=7, y=w806) -> (x = y?=w804:bool)
                  n281 = And(x=w804, y=w803) -> (x .and. y?=w801:bool)
                  n282 = case shown="True" w802 {
                    tunnel: w801 -> [w812 w814]
                    tunnel: [w812 w813] -> w800
                    frame False {
                    }
                    frame True {
                      n283 = Not(x=w814) -> (.not. x?=w813:bool)
                    }
                  }
                  n284 = Select(t=0.0, s=w800, f=100.0) -> (s? t:f=w811:dbl)
                }
                frame True {
                  w823 = 100.0  # Max
                  w824 = 0.0  # Min
                  n285 = call "PID.vi"("Present Value"=w820, "Previous Scan Value"=w815, "Setpoint"=w821) -> ("Dem Output"=w822:dbl)
                  n286 = In Range and Coerce(upper limit=w823, x=w822, lower limit=w824) -> (coerced(x)=w819:dbl)  [unwired: 1 out]
                  n287 = call "Remember_value.vi"("Mode"=Remember_value_mode."Read and Write", "Input Value"=w818, "Ch name"=w817) -> ()  [unwired: 1 out]
                }
              }
            }
          }
        }
        frame "EnFlo_Tunnel:Hydrosonic:Integral" {
          n288 = Build Array("EnFlo_Tunnel:Usonic Fixed:Velocity", "Hydrosonic:Transducer:Setting") -> (w834:string[])
          n289 = call "Read_Earlier_Channels.vi"("Present scan array"=w835, "Ch names"=w833, "Desired Channels"=w834) -> ("Scan comments"=w827:string, "Index 0"=w832:dbl, "Index 1"=w826:dbl)  [unwired: 3 out]
          n290 = Greater?(x=w832, y=0.5) -> (0:w830:bool)
          n291 = case shown="True" w830 {
            tunnel: w829 -> [w838 w846]
            tunnel: [w838 w845] -> w828
            tunnel: w826 -> [_ w844]
            tunnel: w825 -> [_ w843]
            frame False {
            }
            frame True {
              w841 = 8640000.0  # Seconds per day x 100
              n292 = Multiply(x=w844, y=w843) -> (x*y=w842:dbl)
              n293 = Divide(x=w842, y=w841) -> (x/y=w840:dbl)
              n294 = Not A Number/Path/Refnum?(number/path/refnum=w840) -> (NaN/Path/Refnum?=w839:bool)
              n295 = case shown="False" w839 {
                tunnel: w846 -> [w849 w850]
                tunnel: [w848 w850] -> w845
                tunnel: w840 -> [w847 _]
                frame False {
                  n296 = Add(x=w847, y=w849) -> (x+y=w848:dbl)
                }
                frame True {
                }
              }
            }
          }
        }
        frame "EnFlo_Tunnel:Days Run at:2.5m/s" {
          n297 = Build Array("EnFlo_Tunnel:Usonic Fixed:Velocity") -> (w859:string[])
          n298 = call "Read_Earlier_Channels.vi"("Present scan array"=w860, "Ch names"=w858, "Desired Channels"=w859) -> ("Scan comments"=w853:string, "Index 0"=w851:dbl)  [unwired: 4 out]
          n299 = Greater?(x=w851, y=0.5) -> (0:w856:bool)
          n300 = case shown="True" w856 {
            tunnel: w855 -> [w862 w870]
            tunnel: [w862 w869] -> w854
            tunnel: w851 -> [_ w868]
            tunnel: w852 -> [_ w867]
            frame False {
            }
            frame True {
              w865 = 216000.0  # Seconds per day x 2.5
              n301 = Multiply(x=w868, y=w867) -> (x*y=w866:dbl)
              n302 = Divide(x=w866, y=w865) -> (x/y=w864:dbl)
              n303 = Not A Number/Path/Refnum?(number/path/refnum=w864) -> (NaN/Path/Refnum?=w863:bool)
              n304 = case shown="True" w863 {
                tunnel: w870 -> [w873 w874]
                tunnel: [w872 w874] -> w869
                tunnel: w864 -> [w871 _]
                frame False {
                  n305 = Add(x=w871, y=w873) -> (x+y=w872:dbl)
                }
                frame True {
                }
              }
            }
          }
        }
        frame "Complete:Scan:Period" {
          n306 = while {
            tunnel: [w884] -> w877
            tunnel: [w891] -> w879
            shift-left: _ -> [w891]
            shift-right: [w892] -> w880
            tunnel: w876 -> [w888]
            tunnel: [w883] -> w875
            stop <- FALSE continue-if-true
            w883 = 10.0 ("Averaging time (mins)")
            n307 = Build Array(w888) -> (w887:string[])
            n308 = call "Get_Channel_averages.vi"("Desired Ch Names"=w887, "Averaging time (mins)"=w883) -> ("number"=w886:dbl[])  [unwired: 1 in, 2 out]
            n309 = Index Array(array=w886, index=0) -> (element=w884:dbl)
            n310 = Greater?(x=w884, y=20.0) -> (0:w892:bool)
          }
          n311 = Compound Arithmetic op=AND(w880, invert w879) -> (w878:bool)
          n312 = case shown="True" w878 {
            tunnel: w877 -> [_ w898]
            tunnel: w875 -> [_ w893]
            frame False {
            }
            frame True {
              n313 = Format Into String(format string="Warning! The average scan period on the ADAM Scan table is %.1f seconds over the last %d minutes." ("Format String"), w898, w893) -> (resulting string=w896:string)  [unwired: 2 in, 1 out]
              n314 = call "Server_Emails.vi"("Message"=w896, "Contact All clients?"=TRUE, "Subject"="Scan Period") -> ()  [unwired: 2 in, 3 out]
            }
          }
        }
        frame "GMU:Source:Est Time" {
          # "NaN's"
          # "Est?"
          # "Inband?"
          n315 = stacked-sequence {
            seq-local: [w905 _ _ _] -> [_ _ w952 _]
            seq-local: [_ w917 _ _] -> [_ _ w949 _]
            seq-local: [_ w918 _ _] -> [_ _ w947 _]
            seq-local: [_ _ w954 _] -> [_ _ _ w970]
            seq-local: [w909 _ _ _] -> [_ _ w951 _]
            seq-local: [_ w916 _ _] -> [_ _ _ w966]
            tunnel: w904 -> [w911 w919 w957 _]
            tunnel: w903 -> [w910 w920 w958 _]
            tunnel: [_ _ w950 _] -> w902
            tunnel: [_ _ _ w969] -> w901
            tunnel: w900 -> [_ _ _ w968]
            tunnel: w899 -> [_ _ _ w967]
            frame #0 {
              n316 = Build Array("GMU:Source:Density Ratio", "GMU:Source:Dem Strength", "GMU:Source:Dem Q") -> (w912:string[])
              n317 = call "Read_Earlier_Channels.vi"("Present scan array"=w910, "Ch names"=w911, "Desired Channels"=w912) -> ("Scan comments"=w909:string, "Index 0"=w908:dbl, "Index 1"=w907:dbl, "Index 2"=w906:dbl)  [unwired: 2 out]
              n318 = Build Array(w908, w907, w906) -> (w905:dbl[])
            }
            frame #1 {
              n319 = for {
                N: 2 -> [_]
                tunnel: w920 -> [w930]
                tunnel: w919 -> [w931]
                tunnel: [w929] -> w917 mode=indexing
                tunnel: [w936] -> w918 mode=indexing
                tunnel: [w935] -> w916 mode=indexing
                i -> [w941]
                w940 = 23.0  # %
                n320 = case shown="1" w941 {
                  tunnel: ["GMU:Source:Meas Q" "GMU:Source:Meas Strength"] -> w934
                  tunnel: ["GMU:Source:Dem Q" "GMU:Source:Dem Strength"] -> w933
                  frame 0, Default {
                  }
                  frame 1 {
                  }
                }
                n321 = Build Array(w933, w934) -> (w932:string[])
                n322 = call "Read_Earlier_Channels.vi"("Present scan array"=w930, "Ch names"=w931, "Desired Channels"=w932) -> ("Scan comments"=w929:string, "Index 0"=w927:dbl, "Index 1"=w928:dbl)  [unwired: 3 out]
                n323 = Not A Number/Path/Refnum?(number/path/refnum=w928) -> (NaN/Path/Refnum?=w935:bool)
                n324 = Subtract(x=w928, y=w927) -> (x-y=w926:dbl)
                n325 = Greater Than 0?(x=w927) -> (x > 0?=w937:bool)
                n326 = Less?(x=w926, y=0.05) -> (x < y?=w923:bool)
                n327 = call "In_Range_check.vi"("%"=w940, "Mode"=In_Range."%", "Value"=w928, "Setpoint"=w927) -> ("In Range"=w924:bool)  [unwired: 1 in, 2 out]
                n328 = Or(x=w924, y=w923) -> (x .or. y?=w922:bool)
                n329 = And(x=w922, y=w937) -> (x .and. y?=w938:bool)
                n330 = Compound Arithmetic op=OR(w938, invert w937, w935) -> (w936:bool)
              }
            }
            frame #2 {
              n331 = while {
                tunnel: [w965] -> w953
                tunnel: w952 -> [w964]
                shift-left: _ -> [w965]
                shift-right: [w964] -> _
                stop <- FALSE continue-if-true
              }
              n332 = Equal?(x=w952, y=w953) -> (x = y?=w959:bool)
              n333 = call "Read_value_of_earlier_Ch.vi"("Desired Ch to Read"="GMU:Source:Dem Q", "Ch names"=w957, "Present scan array"=w958) -> ("Value"=w955:dbl)  [unwired: 1 in, 1 out]
              n334 = Greater Than 0?(x=w955) -> (x > 0?=w962:bool)
              n335 = And Array Elements(Boolean array=w947) -> (logical AND=w946:bool)
              n336 = Select(t=w946, s=w962, f=TRUE) -> (s? t:f=w960:bool)
              n337 = Compound Arithmetic op=AND(w959, w960) -> (w954:bool)
              n338 = Concatenate Strings(w949) -> (w948:string)
              n339 = Concatenate Strings(w948, w951) -> (w950:string)
            }
            frame #3 {
              n340 = case shown="True" w970 {
                tunnel: [0.0 w972] -> w969
                tunnel: w968 -> [_ w977]
                tunnel: w967 -> [_ w973]
                tunnel: w966 -> [_ w976]
                frame False {
                }
                frame True {
                  n341 = Or Array Elements(Boolean array=w976) -> (logical OR=w975:bool)
                  n342 = Add(x=w977, y=w973) -> (x+y=w974:dbl)
                  n343 = Select(t=w973, s=w975, f=w974) -> (s? t:f=w972:dbl)
                }
              }
            }
          }
        }
      }
    }
    frame "Hold Value" {
    }
    frame "Read A" {
      n344 = Unbundle By Name(w981) -> ("A"=w980:dbl)
    }
    frame "Read Ch" {
      n345 = Unbundle By Name(w986) -> ("String"=w983:string)
      n346 = call "Read_value_of_earlier_Ch.vi"("Desired Ch to Read"=w983, "Ch names"=w987, "Present scan array"=w988) -> ("Value"=w984:dbl, "Scan comment"=w985:string)  [unwired: 1 in]
    }
    frame "Coded" {
    }
    frame "Client Info" {
      n347 = global read "ADAM_Global.vi" "Client State Array"() -> (w1003:T15[])
      n348 = call "Split_Ch_name.vi"("Ch name"=w997) -> ("Top level"=w995:string, "Low level"=w993:string)  [unwired: 1 out]
      n349 = Equal?(x="Status" ("Substring"), y=w995) -> (x = y?=w994:bool)
      n350 = Select(t=w993, s=w994, f="") -> (s? t:f=w991:string)
      n351 = for {
        tunnel: w1003 -> [w1012] mode=indexing
        tunnel: [w1011] -> w1004 mode=indexing
        n352 = Unbundle By Name(w1012) -> ("Client Name"=w1011:string)
      }
      n353 = Search 1D Array(1D array=w1004, element=w991) -> (index of element=w999:i32)  [unwired: 1 out]
      n354 = Less Than 0?(x=w999) -> (x < 0?=w998:bool)
      n355 = Index Array(array=w1003, index=w999) -> (element=w1002:T15)
      n356 = case shown="False" w998 {
        tunnel: w1002 -> [w1007 _]
        tunnel: w991 -> [w1006 w1009]
        tunnel: [w1005 w1008] -> w1001
        frame False {
          n357 = call "Get_Client_Status_string.vi"("Client State Cluster"=w1007, "Client Name"=w1006) -> ("Code Value"=w1005:dbl)  [unwired: 1 in]
        }
        frame True {
          w1008 = 7.0 ("Code Value")
          n358 = call "Remember_value.vi"("Mode"=Remember_value_mode."Read and Write", "Input Value"=w1008, "Ch name"=w1009) -> ()  [unwired: 1 out]
        }
      }
    }
    frame "Web Client" {
      w1022 = 7200.0  # 2 Hours in Seconds
      n359 = Concatenate Strings(w1031, ":Last read" ("Substring")) -> (w1029:string)
      n360 = call "Remember_value.vi"("Mode"=Remember_value_mode."Read only", "Ch name"=w1029) -> ("Output Value"=w1028:dbl)  [unwired: 1 in]
      n361 = Not A Number/Path/Refnum?(number/path/refnum=w1028) -> (NaN/Path/Refnum?=w1026:bool)
      n362 = Get Date/Time In Seconds() -> (seconds since 1Jan1904=w1021:timestamp)
      n363 = To Double Precision Float(number=w1021) -> (double precision float=w1019:dbl)
      n364 = Subtract(x=w1019, y=w1028) -> (x-y=w1034:dbl)
      n365 = Greater?(x=w1034, y=1800.0) -> (0:w1027:bool)
      n366 = Or(x=w1027, y=w1026) -> (x .or. y?=w1013:bool)
      n367 = case shown="True" w1013 {
        frame False {
        }
        frame True {
          n368 = global read "Constants_global.vi" "EnFlo SW Folder"() -> (w1037:path)
          n369 = Build Path(base path=w1037, name or relative path=path "ADAM Server/Sub VI's/Web_Client.vi") -> (appended path=w1036:path)
          n370 = Open VI Reference(vi path=w1036) -> (vi reference=w1041:refnum<vi>, error out=w1042:errorcluster)  [unwired: 1 in, 4 out]
          n371 = property class="VI"(reference=w1041, error in=w1042) -> (reference out=w1044:refnum<vi>, error out=w1045:errorcluster, "Front Panel Window:Open"=w1043:bool)
          n372 = case shown="False" w1043 {
            tunnel: w1044 -> [w1051 w1054]
            tunnel: w1045 -> [w1050 w1053]
            tunnel: [w1049 w1054] -> w1046
            tunnel: [w1048 w1053] -> w1047
            frame False {
              n373 = property class="VI"(reference=w1051, error in=w1050, "Front Panel Window:Open"=TRUE) -> (reference out=w1049:refnum<vi>, error out=w1048:errorcluster)
            }
            frame True {
            }
          }
          n374 = invoke class="VI" method="Run VI"(reference=w1046, error in=w1047, "Wait until done"=FALSE, "Auto Dispose Ref"=TRUE) -> ()  [unwired: 1 in, 5 out]
        }
      }
      n375 = Concatenate Strings(w1031, ":value time" ("Substring")) -> (w1015:string)
      n376 = call "Remember_value.vi"("Mode"=Remember_value_mode."Read only", "Ch name"=w1031) -> ("Output Value"=w1035:dbl)  [unwired: 1 in]
      n377 = call "Remember_value.vi"("Mode"=Remember_value_mode."Read only", "Ch name"=w1015) -> ("Output Value"=w1020:dbl)  [unwired: 1 in]
      n378 = Subtract(x=w1019, y=w1020) -> (x-y=w1018:dbl)
      n379 = Greater?(x=w1018, y=w1022) -> (0:w1025:bool)
      n380 = case shown="True" w1025 {
        tunnel: w1018 -> [_ w1060]
        tunnel: 3600.0 ("y") -> [_ w1059]
        tunnel: ["" w1057] -> w1024
        frame False {
        }
        frame True {
          n381 = Divide(x=w1060, y=w1059) -> (x/y=w1056:dbl)
          n382 = Format Into String(format string="Value is %d hours old." ("Format String"), w1056) -> (resulting string=w1057:string)  [unwired: 2 in, 1 out]
        }
      }
    }
    frame "X10" {
      (unwired) 1 items=["-----", "A", "B", "C", "D", "E", "F", "G", "H", "I", "J", "K", "L", "M", "N", "O", "P"] ("House Code")
      n383 = Greater Than 0?(x=w1065) -> (x > 0?=w1064:bool)
      n384 = Unbundle By Name(w1070) -> ("Port Name"=w1067:string, "Main"=w1068:i32, "Ch."=w1069:i32)
      n385 = call "X10control.vi"("Port Name"=w1067, "Power Request (ON)"=w1064, "House Code"=w1068, "Unit No."=w1069) -> ()  [unwired: 6 out]
      n386 = Select(t=1.0, s=w1064, f=0.0) -> (s? t:f=w1061:dbl)
    }
    frame "LPA" {
      # "LPA was, IIRC, a serially-polled weighing platform we rented at Surrey for Athena Scaperdas' project at Atkins to weigh a helicopter with rotor running. \nTo add to the fun, it was RS232, so to make it addressable it was polled through an addressable ADAM 485-232 module"
      n387 = call "LPA400_get_rdg.vi"("Channel Name"=w1073, "Address"=w1074) -> ("Output"=w1071:dbl, "Status note"=w1072:string)  [unwired: 4 out]
    }
    frame "ScanPacer" {
      # "Uses a metronome to slow an otherwise over-fast scan table"
      n388 = call "ADAMPacer.vi"("Ch Description"=w1077) -> ("Scan comment"=w1075:string, "Output"=w1076:dbl)  [unwired: 7 in]
    }
    frame "Test" {
      w1081 = 0.0005  # y
      n389 = Get Date/Time In Seconds() -> (seconds since 1Jan1904=w1078:timestamp)
      n390 = To Double Precision Float(number=w1078) -> (double precision float=w1083:dbl)
      n391 = Subtract(x=w1083, y=2969882881.0) -> (x-y=w1082:dbl)
      n392 = Multiply(x=w1082, y=w1081) -> (x*y=w1079:dbl)
      n393 = Random Number (0-1)() -> (number: 0 to 1=w1080:dbl)
      n394 = Add(x=w1080, y=w1079) -> (x+y=w1086:dbl)
    }
    frame "Oops", Default {
    }
  }
  "Output" <- w8
  "Scan comment" <- w5
